vi "test1-HexStr conversion.vi"(8 "error in (no error)":errorcluster, 11 "TestCase in":refnum<class "testcase-CSMArgument.lvclass">) -> (0 "error out":errorcluster, 3 "TestCase out":refnum<class "testcase-CSMArgument.lvclass">)   [LabVIEW 2017, in "testcase-CSMArgument.lvclass"]
uses:
  testcase-CSMArgument.lvclass
  src/user.lib/_NEVSTOP/Communicable State Machine(CSM)/_Shared/Trim Single-line Text.vi
  <vilib>/addons/_JKI Toolkits/VI Tester/TestCase.llb/TestCase.lvclass
  src/user.lib/_NEVSTOP/Communicable State Machine(CSM)/Communicable State Machine.lvlib
  src/user.lib/_NEVSTOP/Communicable State Machine(CSM)/_Shared/CSM Shared.lvlib
  C:/Program Files (x86)/National Instruments/LabVIEW 2017/vi.lib/addons/_JKI Toolkits/VI Tester/TestCase.llb/TestCase.lvclass
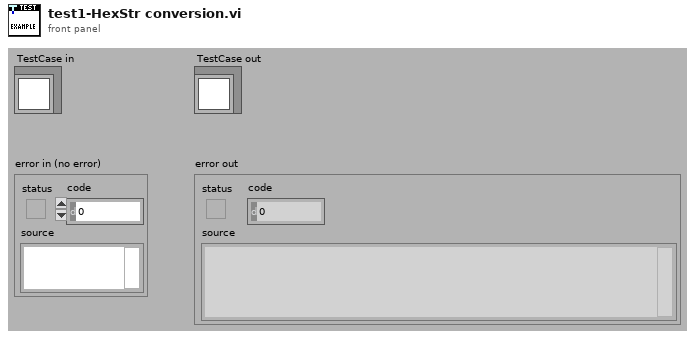
[diagram p1: front panel]
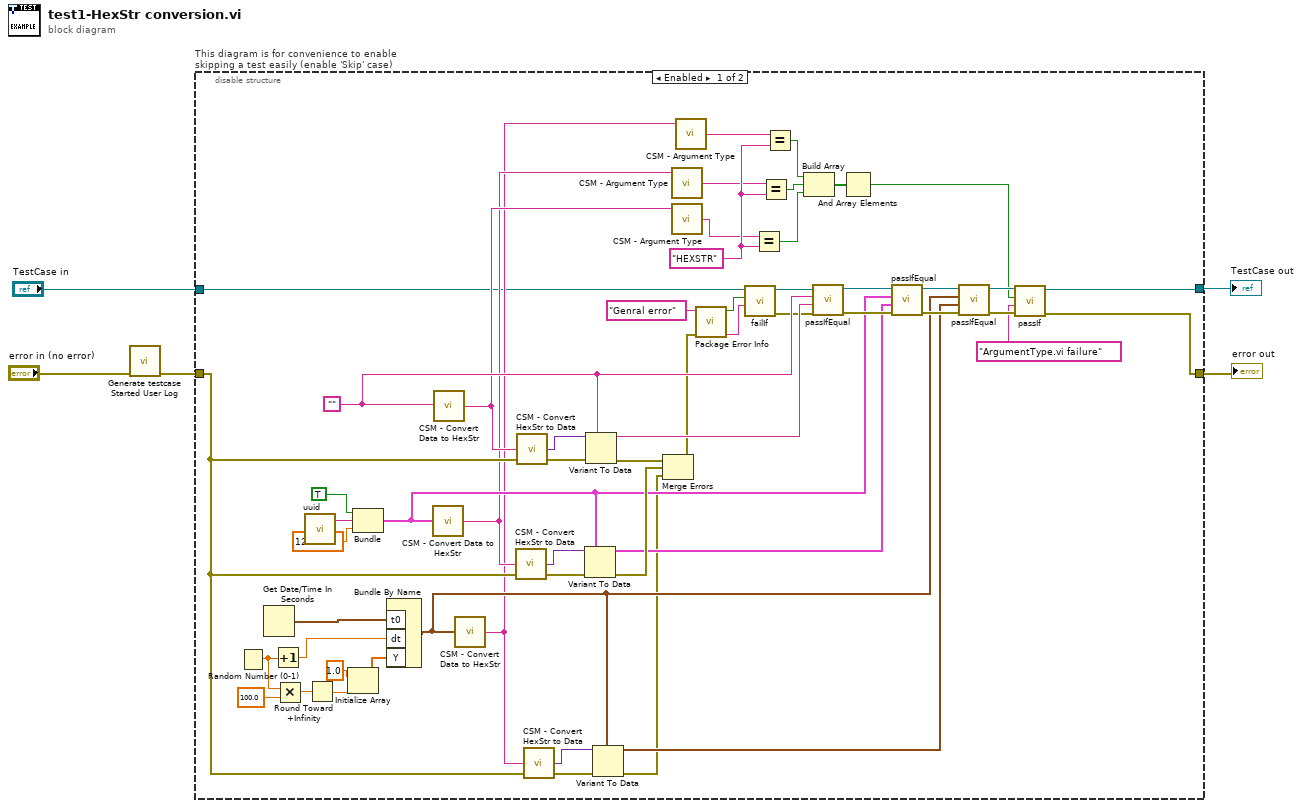
[diagram p0: block diagram]
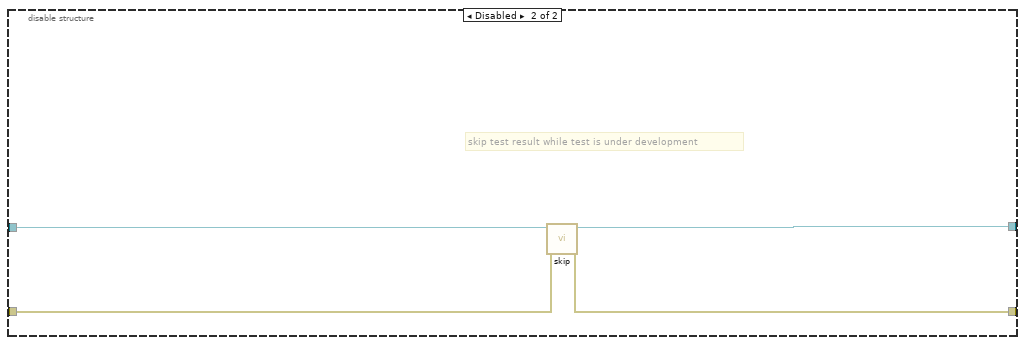
[diagram p2: hidden frame]
diagram:
  n1 = call "Generate testcase Started User Log.vi"("Error In"="error in (no error)") -> ("error out"=w1:errorcluster)  [unwired: 10 in]
  n2 = disable-structure "This diagram is for convenience to enable skipping a test easily (enable 'Skip' case)" shown="Enabled" {
    disable-tunnel: "TestCase in" -> [w12 w64]
    disable-tunnel: [w20 w62] -> w2
    disable-tunnel: [w18 w63] -> w4
    disable-tunnel: w1 -> [w43 w61]
    frame Enabled {
      w26 = "HEXSTR"
      w54 = ""
      n3 = Random Number (0-1)() -> (number: 0 to 1=w39:dbl)
      n4 = Get Date/Time In Seconds() -> (seconds since 1Jan1904=w42:timestamp)
      n5 = Increment(x=w39) -> (x+1=w41:dbl)
      n6 = Multiply(x=w39, y=100.0) -> (x*y=w37:dbl)
      n7 = call "uuid.vi"() -> ("UUID"=w59:string)  [unwired: 11 in]
      n8 = Round Toward +Infinity(x=w37) -> (ceil(x): smallest int >= x=w36:dbl)
      n9 = Initialize Array(1.0 ("element"), w36) -> (w35:dbl[])
      n10 = Bundle(TRUE, "UUID"=w59, 123.456) -> (w47:cluster{bool, "UUID":string, dbl})  [unwired: 1 in]
      n11 = Bundle By Name("t0"=w42, "dt"=w41, "Y"=w35) -> (w32:waveform(dbl))  [unwired: 1 in]
      n12 = call "CSM - Convert Data to HexStr.vi"("Variant"=w47) -> ("HEX String (0-9,A-F)"=w28:string)  [unwired: 8 in]
      n13 = call "CSM - Convert Data to HexStr.vi"("Variant"=w54) -> ("HEX String (0-9,A-F)"=w29:string)  [unwired: 8 in]
      n14 = call "CSM - Convert Data to HexStr.vi"("Variant"=w32) -> ("HEX String (0-9,A-F)"=w27:string)  [unwired: 8 in]
      n15 = call "CSM - Convert HexStr to Data.vi"("HEX String"=w28, "error in (no error)"=w43) -> ("Variant"=w50:variant, "error out"=w52:errorcluster)  [unwired: 6 in]
      n16 = call "CSM - Convert HexStr to Data.vi"("HEX String"=w29, "error in (no error)"=w43) -> ("Variant"=w55:variant, "error out"=w57:errorcluster)  [unwired: 6 in]
      n17 = call "CSM - Convert HexStr to Data.vi"("HEX String"=w27, "error in (no error)"=w43) -> ("Variant"=w45:variant, "error out"=w44:errorcluster)  [unwired: 6 in]
      n18 = Variant To Data(error in=w52, type=w47, Variant=w50) -> (data=w46:cluster{bool, "UUID":string, dbl}, error out=w51:errorcluster)
      n19 = Variant To Data(error in=w57, type=w54, Variant=w55) -> (data=w53:string, error out=w56:errorcluster)
      n20 = Variant To Data(error in=w44, type=w32, Variant=w45) -> (data=w31:waveform(dbl), error out=w30:errorcluster)
      n21 = Merge Errors(w56, w51, w30) -> (w6:errorcluster)
      n22 = call "CSM - Argument Type.vi"("Arguments"=w28) -> ("Argument Type"=w16:string)  [unwired: 3 in, 1 out]
      n23 = call "CSM - Argument Type.vi"("Arguments"=w29) -> ("Argument Type"=w15:string)  [unwired: 3 in, 1 out]
      n24 = call "CSM - Argument Type.vi"("Arguments"=w27) -> ("Argument Type"=w13:string)  [unwired: 3 in, 1 out]
      n25 = call "Package Error Info.vi"("error in"=w6, "String in"="Genral error") -> ("packed error info out"=w8:string, "error status"=w9:bool)  [unwired: 8 in]
      n26 = call-dynamic "failIf.vi"("message (\"\")"=w8, "fail"=w9, "TestCase in"=w12) -> ("error out"=w10:errorcluster, "TestCase out"=w11:refnum<class "testcase-CSMArgument.lvclass">)  [unwired: 7 in]
      n27 = Equal?(x=w15, y=w26) -> (x = y?=w23:bool)
      n28 = Equal?(x=w16, y=w26) -> (x = y?=w25:bool)
      n29 = Equal?(x=w13, y=w26) -> (x = y?=w24:bool)
      n30 = Build Array(w24, w25, w23) -> (w22:bool[])
      n31 = call-dynamic "passIfEqual.vi"("error in (no error)"=w10, "y"=w53, "x"=w54, "TestCase in"=w11) -> ("error out"=w48:errorcluster, "TestCase out"=w49:refnum<class "testcase-CSMArgument.lvclass">)  [unwired: 6 in]
      n32 = And Array Elements(Boolean array=w22) -> (logical AND=w17:bool)
      n33 = call-dynamic "passIfEqual.vi"("error in (no error)"=w48, "y"=w46, "x"=w47, "TestCase in"=w49) -> ("error out"=w33:errorcluster, "TestCase out"=w34:refnum<class "testcase-CSMArgument.lvclass">)  [unwired: 6 in]
      n34 = call-dynamic "passIfEqual.vi"("error in (no error)"=w33, "y"=w31, "x"=w32, "TestCase in"=w34) -> ("error out"=w19:errorcluster, "TestCase out"=w21:refnum<class "testcase-CSMArgument.lvclass">)  [unwired: 6 in]
      n35 = call-dynamic "passIf.vi"("error in (no error)"=w19, "message (\"\")"="ArgumentType.vi failure", "pass"=w17, "TestCase in"=w21) -> ("error out"=w18:errorcluster, "TestCase out"=w20:refnum<class "testcase-CSMArgument.lvclass">)  [unwired: 6 in]
    }
    frame Disabled {
      # "skip test result while test is under development"
      n36 = call <vilib>:"skip.vi"("error in (no error)"=w61, "TestCase in"=w64) -> ("error out"=w63:errorcluster, "TestCase out"=w62:refnum<class "testcase-CSMArgument.lvclass">)  [unwired: 8 in]
    }
  }
  "error out" <- w4
  "TestCase out" <- w2
